vi "生成雷区.vi"(9 "雷数":dbl, 10 "firstPT":cluster{"行":dbl, "列":dbl}, 11 "输入":dbl[][](array[numeric])) -> (3 "输出":dbl[][](array[numeric]))   [LabVIEW 2023]
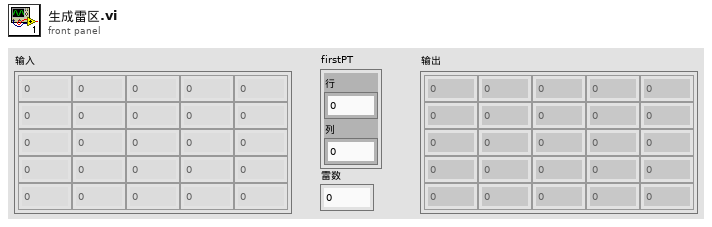
[diagram p1: front panel]
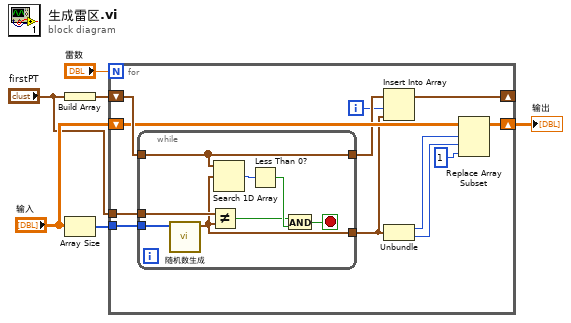
[diagram p0: block diagram]
diagram:
  n1 = Build Array("firstPT") -> (w1:cluster{"行":dbl, "列":dbl}[])
  n2 = Array Size(array="输入") -> (size(s)=w4:i32[])
  n3 = for {
    N: "雷数" -> [_]
    shift-right: [w11] -> w6
    shift-left: "输入" -> [w15]
    tunnel: "firstPT" -> [w18]
    tunnel: w4 -> [w17]
    shift-right: [w9] -> _
    shift-left: w1 -> [w16]
    i -> [w7]
    n4 = while {
      tunnel: w18 -> [w24]
      tunnel: w17 -> [w26]
      tunnel: w16 -> [w19]
      tunnel: [w20] -> w8
      tunnel: [w19] -> w10
      stop <- w21 stop-if-true
      n5 = call "随机数生成.vi"("数组"=w26) -> ("簇"=w20:cluster{"行":i32, "列":i32})  [unwired: 10 in]
      n6 = Not Equal?(x=w24, y=w20) -> (x != y?=w22:bool)
      n7 = Search 1D Array(1D array=w19, element=w20) -> (index of element=w25:i32)  [unwired: 1 in]
      n8 = Less Than 0?(x=w25) -> (x < 0?=w23:bool)
      n9 = And(x=w22, y=w23) -> (x .and. y?=w21:bool)
    }
    n10 = Insert Into Array(array=w10, index=w7, new element=w8) -> (w9:cluster{"行":dbl, "列":dbl}[])
    n11 = Unbundle(w8) -> ("行"=w14:i32, "列"=w13:i32)
    n12 = Replace Array Subset(array=w15, new element=1 ("数值 2"), index (row)=w14, index (col)=w13) -> (w11:dbl[][])
  }
  "输出" <- w6
